vi "WriteInputMap.vi"(8 "Error In":errorcluster, 10 "Input Map":map{string, bool}(c390), 11 "object in":refnum<class "Conjunction.lvclass">) -> (0 "Error Out":errorcluster, 3 "object out":refnum<class "Conjunction.lvclass">)   [LabVIEW 2021, in "Conjunction.lvclass"]
uses:
  Conjunction.lvclass
  Conjunction.lvclass/Conjunction.ctl
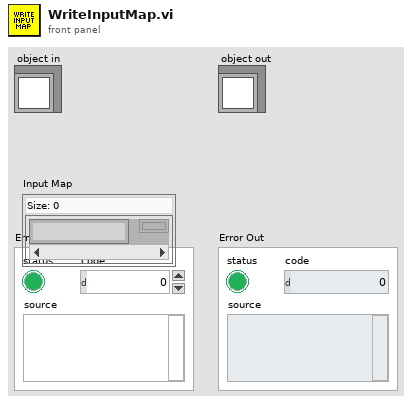
[diagram p1: front panel]
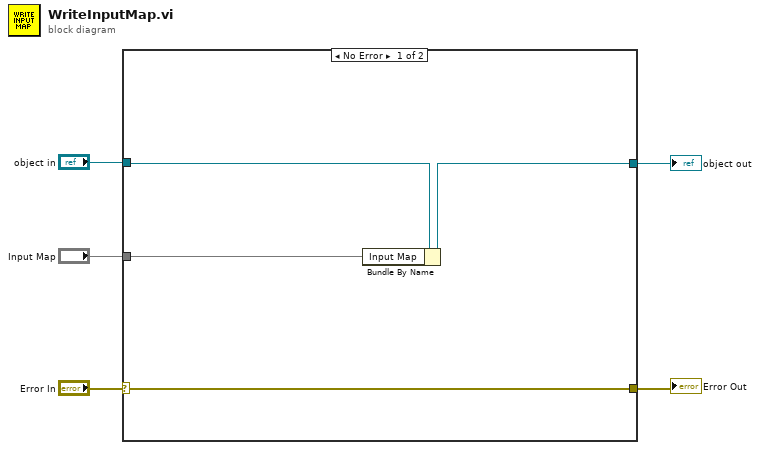
[diagram p0: block diagram]
diagram:
  n1 = case shown="No Error" "Error In" {
    selector: "Error In" -> [w8 w11]
    tunnel: [w8 w11] -> w4
    tunnel: [w6 w10] -> w2
    tunnel: "object in" -> [w7 w10]
    tunnel: "Input Map" -> [w9 _]
    frame No Error {
      n2 = Bundle By Name(cluster=w7, "Input Map"=w9) -> (w6:refnum<class "Conjunction.lvclass">)
    }
    frame Error {
    }
  }
  "Error Out" <- w4
  "object out" <- w2
